vi "Read Mapping offset.vi"(8 "error in (no error)":errorcluster, 11 "Mapping params in":refnum<class "CV-Mapping.lvclass">) -> (0 "error out":errorcluster, 2 "Mapping off-set":dbl caption="Mapping off-set [s]", 3 "Mapping params out":refnum<class "CV-Mapping.lvclass">)   [LabVIEW 2013, in "CameraVision.lvlib" / "CV-Mapping.lvclass"]
uses:
  CV-Mapping.lvclass
  CV-Mapping.lvclass/CV-Mapping.ctl
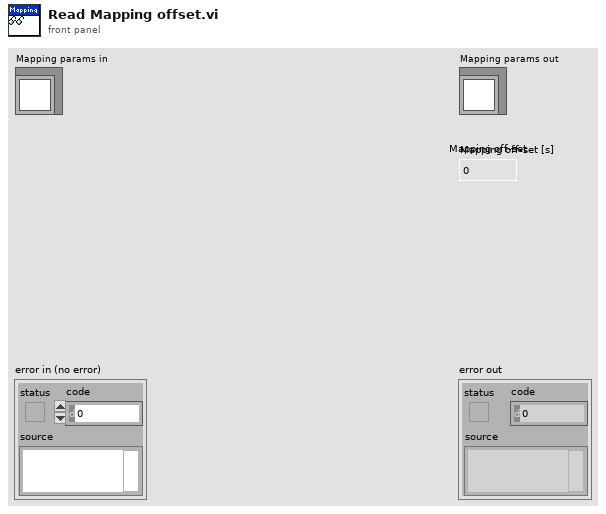
[diagram p1: front panel]
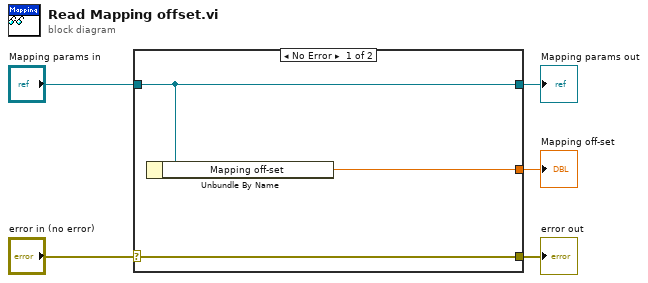
[diagram p0: block diagram]
diagram:
  n1 = case shown="No Error" "error in (no error)" {
    selector: "error in (no error)" -> [w8 w9]
    tunnel: [w8 w9] -> w4
    tunnel: [w7 w10] -> w2
    tunnel: "Mapping params in" -> [w7 w10]
    tunnel: [w6 _] -> w1
    frame No Error {
      n2 = Unbundle By Name(w7) -> ("Mapping off-set"=w6:dbl)
    }
    frame Error {
    }
  }
  "error out" <- w4
  "Mapping params out" <- w2
  "Mapping off-set" <- w1
